vi "On Acquire.vi"(4 "Acquisition Status Notifier":refnum<notifier>, 5 "Diagnostics Queue":refnum<queue>, 6 "Force?":bool, 7 "Host Resources":T1, 8 "error in (no error)":errorcluster, 9 "Data Queue":refnum<queue>, 10 "Data Notifier":refnum<notifier>, 11 "Hardware Resources in":T4) -> (0 "error out":errorcluster, 3 "Hardware Resources out":T4)   [LabVIEW 2021, in "Acquisition.lvlib"]
doc: "If the current interval has elapsed, read new data from the data acqusition hardware, post process it, and send it to the 'Data Queue' and 'Data Notifier'.\n\nIf the current interval has not elapsed, calculate the time remaining and send an estimated countdown to 'Acquisition Status Notifier'.\n\nIf 'Force?' is TRUE, ignore the interval and acquire anyway."
uses:
  Acquisition.lvlib
  Hardware Configuration.ctl
  Channel Settings.ctl
  IO Device.ctl
  Sensor Type.ctl
  Interval Timer/Repeat Interval.ctl
  Interval Timer/Interval Length.ctl
  Interval Timer/Interval Token.ctl
  IO Context.ctl
  IO API.ctl
  Acquired Data.ctl
  controls/Acquisition Status.ctl
  support/Message Queue/Message Cluster.ctl
  Host Resources.ctl
  Host Software Package.ctl
  Host IO Resource.ctl
  Interval Timer/Interval Timer.lvlib
  support/Message Queue/Message Queue.lvlib
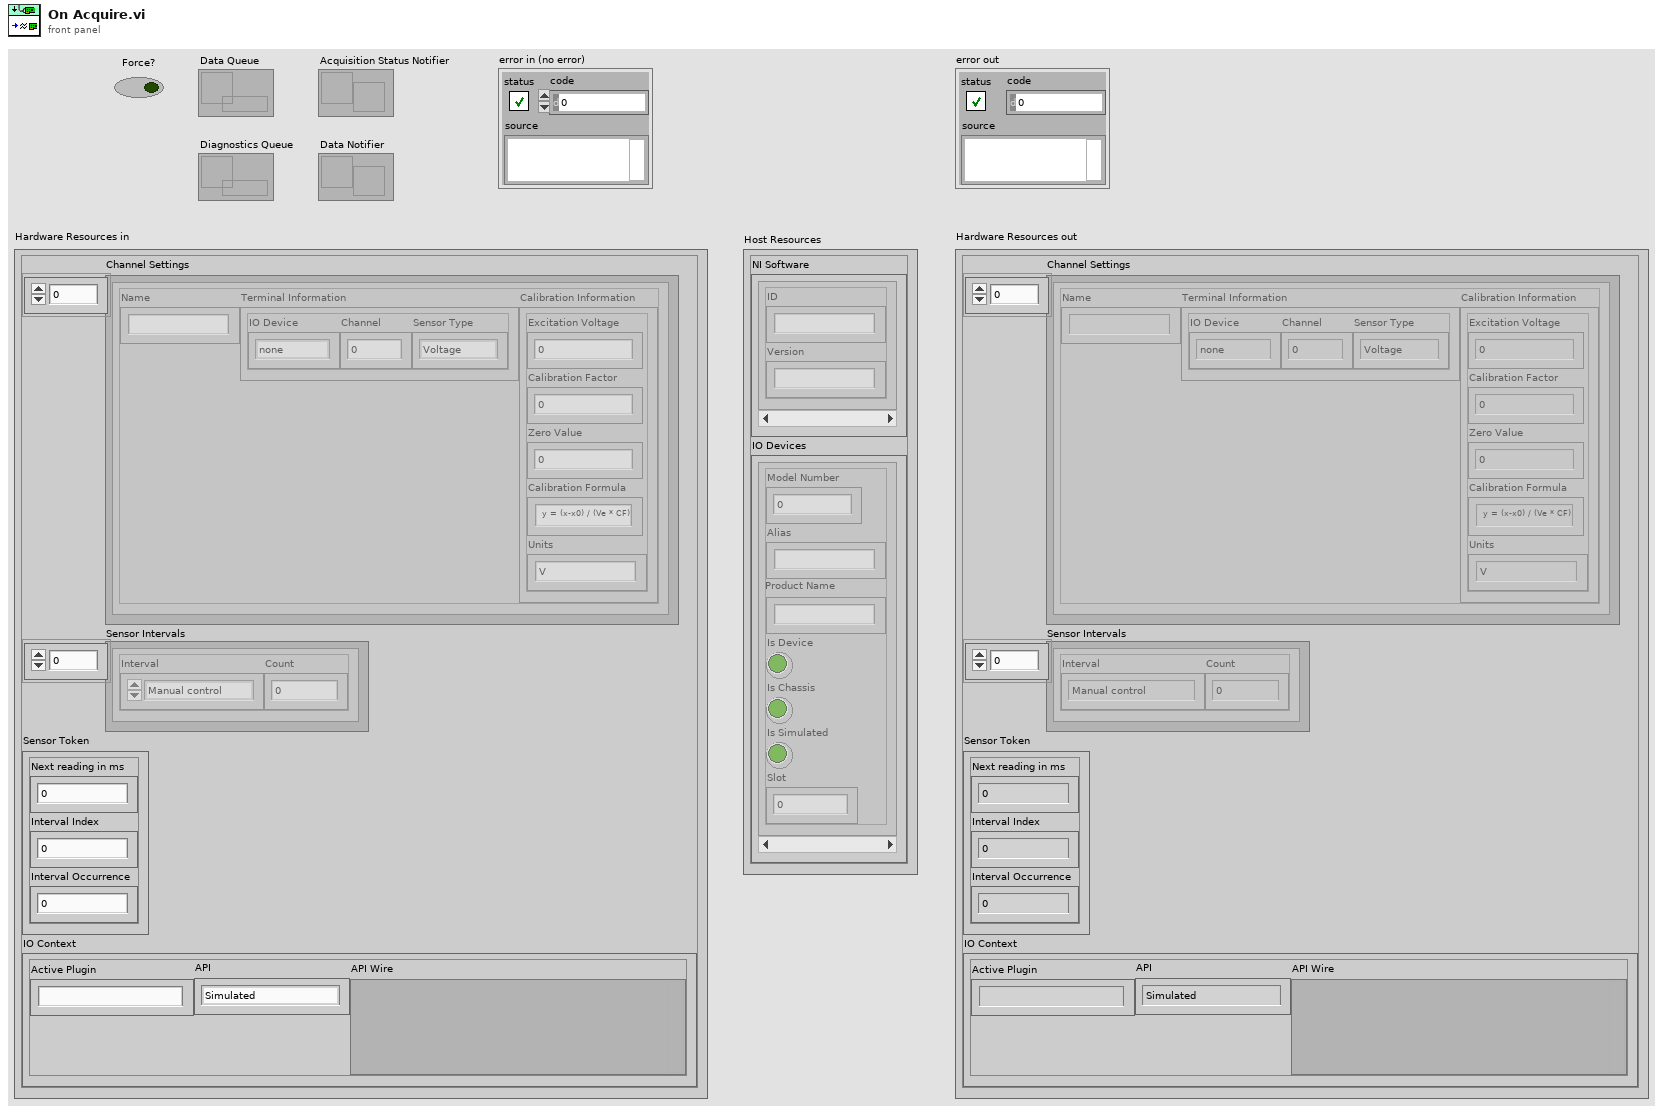
[diagram p1: front panel]
types:
  T1 = typedef "Acquisition.lvlib/Host Resources.ctl" = cluster{"NI Software":T2[], "IO Devices":T3[]}
  T2 = typedef "Acquisition.lvlib/Host Software Package.ctl" = cluster{"ID":string, "Version":string}
  T3 = typedef "Acquisition.lvlib/Host IO Resource.ctl" = cluster{"Model Number":u32, "Alias":string, "Product Name":string, "Is Device":bool, "Is Chassis":bool, "Is Simulated":bool, "Slot":i32}
  T4 = typedef "Acquisition.lvlib/Hardware Configuration.ctl" = cluster{"Channel Settings":T5[], "Sensor Intervals":T8[], "Sensor Token":T10, "IO Context":T11}
  T5 = typedef "Acquisition.lvlib/Channel Settings.ctl" = cluster{"Name":string, "Terminal Information":cluster{"IO Device":T6, "Channel":i32, "Sensor Type":T7}, "Calibration Information":cluster{"Excitation Voltage":dbl, "Calibration Factor":dbl, "Zero Value":dbl, "Calibration Formula":string, "Units":string}}
  T6 = typedef "Acquisition.lvlib/IO Device.ctl" = enum16{"none", "9219", "9401"}
  T7 = typedef "Acquisition.lvlib/Sensor Type.ctl" = enum16{"Voltage", "Load", "Pressure", "Encoder"}
  T8 = typedef "Interval Timer.lvlib/Repeat Interval.ctl" = cluster{"Interval":T9, "Count":i32}
  T9 = typedef "Interval Timer.lvlib/Interval Length.ctl" = enum16{"Manual control", "1 second", "10 seconds", "30 seconds", "60 seconds", "600 seconds", "1200 seconds", "3600 seconds"}
  T10 = typedef "Interval Timer.lvlib/Interval Token.ctl" = cluster{"Next reading in ms":u32, "Interval Index":i32, "Interval Occurrence":i32}
  T11 = typedef "Acquisition.lvlib/IO Context.ctl" = cluster{"Active Plugin":string, "API":T12, "API Wire":variant}
  T12 = typedef "Acquisition.lvlib/IO API.ctl" = enum16{"Simulated", "DAQmx"}
  T13 = typedef "Acquisition.lvlib/Acquired Data.ctl" = cluster{"Waveform Array":waveform(dbl)[]}
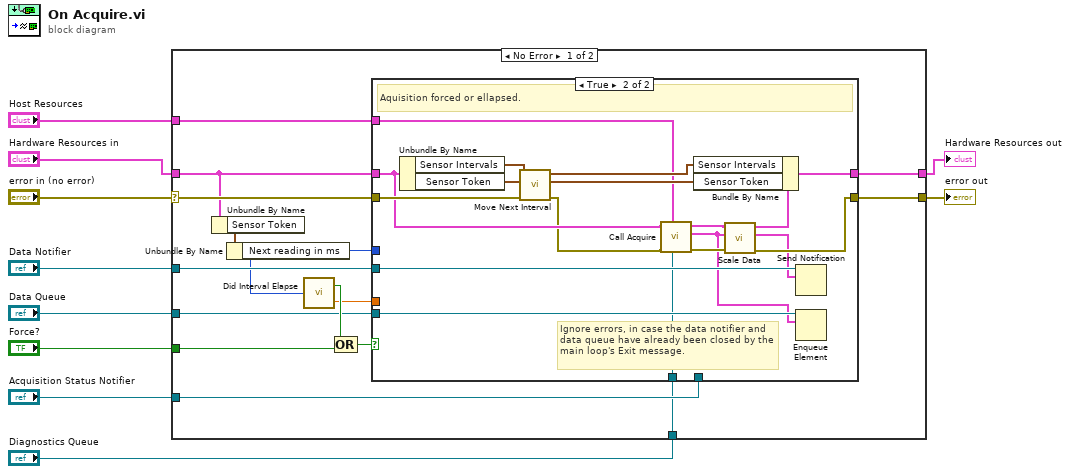
[diagram p0: block diagram]
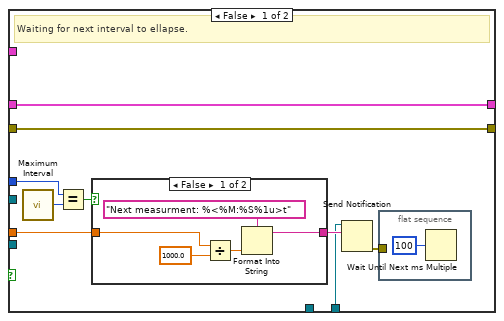
[diagram p2: hidden frame]
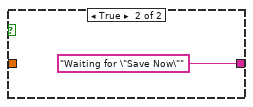
[diagram p3: hidden frame]
diagram:
  n1 = case shown="No Error" "error in (no error)" {
    selector: "error in (no error)" -> [w22 w60]
    tunnel: [w21 w60] -> w9
    tunnel: "Hardware Resources in" -> [w16 w61]
    tunnel: [w15 w61] -> w7
    tunnel: "Data Notifier" -> [w19 _]
    tunnel: "Data Queue" -> [w20 _]
    tunnel: "Force?" -> [w24 _]
    tunnel: "Acquisition Status Notifier" -> [w18 _]
    tunnel: "Host Resources" -> [w12 _]
    tunnel: "Diagnostics Queue" -> [w11 _]
    frame No Error {
      n2 = Unbundle By Name(w16) -> ("Sensor Token"=w13:T10)
      n3 = Unbundle By Name(w13) -> ("Next reading in ms"=w14:u32)
      n4 = call "Did Interval Elapse.vi"("Future time coordinate (ms)"=w14) -> ("ms Until Next"=w17:dbl, "Interval Elapsed?"=w25:bool)  [unwired: 2 in]
      n5 = Compound Arithmetic op=OR(w25, w24) -> (w23:bool)
      n6 = case shown="True" w23 {
        tunnel: w22 -> [w34 w51]
        tunnel: [w34 w50] -> w21
        tunnel: w20 -> [_ w59]
        tunnel: w19 -> [_ w58]
        tunnel: w18 -> [w31 _]
        tunnel: w17 -> [w30 _]
        tunnel: w14 -> [w28 _]
        tunnel: w16 -> [w26 w46]
        tunnel: [w26 w52] -> w15
        tunnel: w12 -> [_ w48]
        tunnel: w11 -> [_ w43]
        frame False {
          # "Waiting for next interval to ellapse."
          n7 = call "Maximum Interval.vi"() -> ("Maximum interval (ms)"=w27:u32)
          n8 = Equal?(x=w28, y=w27) -> (x = y?=w29:bool)
          n9 = case shown="False" w29 {
            tunnel: [w38 "Waiting for \"Save Now\""] -> w33
            tunnel: w30 -> [w37 _]
            frame False {
              n10 = Divide(x=w37, y=1000.0) -> (x/y=w36:dbl)
              n11 = Format Into String(format string="Next measurment: %<%M:%S%1u>t", w36) -> (resulting string=w38:string)  [unwired: 2 in, 1 out]
            }
            frame True {
            }
          }
          n12 = Send Notification(notification=w33, notifier=w31) -> (error out=w32:errorcluster)  [unwired: 1 in, 1 out]
          n13 = flat-sequence {
            tunnel: w32 -> [_]
            frame #0 {
              n14 = Wait Until Next ms Multiple(millisecond multiple=u32 100) -> ()  [unwired: 1 out]
            }
          }
        }
        frame True {
          # "Ignore errors, in case the data notifier and data queue have already been closed by the main loop's Exit message."
          # "Aquisition forced or ellapsed."
          n15 = Unbundle By Name(w46) -> ("Sensor Intervals"=w57:T8[], "Sensor Token"=w56:T10)
          n16 = call "Move Next Interval.vi"("error in"=w51, "Interval Token in"=w56, "Intervals in"=w57) -> ("error out"=w45:errorcluster, "Interval Token out"=w53:T10, "Intervals out"=w54:T8[])  [unwired: 5 in, 1 out]
          n17 = call "Call Acquire.vi"("Diagnostics Queue in"=w43, "Host Resources"=w48, "error in (no error)"=w45, "Hardware Configuration in"=w46) -> ("error out"=w44:errorcluster, "Acquired Data"=w42:T13, "Hardware Configuration out"=w47:T4)  [unwired: 5 in]
          n18 = call "Scale Data.vi"("error in"=w44, "Raw Graph Data"=w42, "Channel Settings in"=w47) -> ("error out"=w50:errorcluster, "Scaled Graph Data"=w49:T13, "Channel Settings out"=w55:T4)  [unwired: 6 in]
          n19 = Bundle By Name(cluster=w55, "Sensor Intervals"=w54, "Sensor Token"=w53) -> (w52:T4)
          n20 = Send Notification(notification=w49, notifier=w58) -> ()  [unwired: 1 in, 2 out]
          n21 = Enqueue Element(queue=w59, element=w42) -> ()  [unwired: 2 in, 3 out]
        }
      }
    }
    frame Error {
    }
  }
  "Hardware Resources out" <- w7
  "error out" <- w9
